vi "RF with WF Sweep plus reference.vi"() -> ()   [LabVIEW 2012]
uses:
  <vilib>/DAQmx/read.llb/DAQmx Read (Counter U32 1Chan 1Samp).vi
  <vilib>/Utility/file.llb/Write To Spreadsheet File (DBL).vi
  <vilib>/DAQmx/miscellaneous.llb/DAQmx Fill In Error Info.vi
  <vilib>/DAQmx/create/channels.llb/DAQmx Create Channel (CI-Count Edges).vi
  <vilib>/DAQmx/create/channels.llb/DAQmx Create Channel (CO-Pulse Generation-Ticks).vi
  <vilib>/DAQmx/configure/timing.llb/DAQmx Timing (Implicit).vi
  <vilib>/DAQmx/configure/timing.llb/DAQmx Timing (Sample Clock).vi
  <resource>/objmgr/daqmx.rc
panel:
  out "Ref":dbl=487.0
  out "Scan":i32=222
  in  "N Scans":i32=100
  out "freq":dbl=349000000.0
  out "RF":dbl=487.0
  out "loop":i32=99
  in  "file path (dialog if empty)":path
  out "Z Position 2":dbl=39.24
  out "Y Position 2":dbl=141.00216667506004
  out "X Position 2":dbl=-28.668339852561274
  in  "CW for tracking":bool
  in  "Y Parameters":T1={"Number of Y Steps"=200, "Max Y (V)"=2.0, "Min Y (V)"=-2.0}
  in  "X":T2={"Number of X Steps"=200, "Max X (V)"=2.0, "Min X (V)"=-2.0}
  in  "Z Position":dbl=39.24
  in  "Y Position":dbl=136.0
  in  "X Position":dbl=-24.0
  in  "Z-track?":bool=TRUE
  out "XY Graph":cluster{dbl[], u32[]}[](graph)
  in  "Freq Max":dbl=350000000.0
  in  "Freq  Step":dbl=1000000.0
  in  "Freq Min":dbl=250000000.0
  in  "power":dbl=-9.0
  in  "stop":bool
  in  "Path to spinapi.dll":path=path "C:/SpinCore/SpinAPI/dll/spinapi64.dll"
  in  "Pulse offset":dbl
  in  "Tau":dbl=5e-07
  in  "RF Pulse":dbl=1e-07
  in  "Rabi Freq":dbl=11750000.0
  in  "MW Delay":dbl=2e-08
  in  "APD signal width":dbl=3e-07
  in  "Signal Delay":dbl=7.6e-07
  in  "AOM Rest time":dbl=1e-06
  in  "AOM Pulse length":dbl=2.5e-06
  in  "N Loop":i32=100000
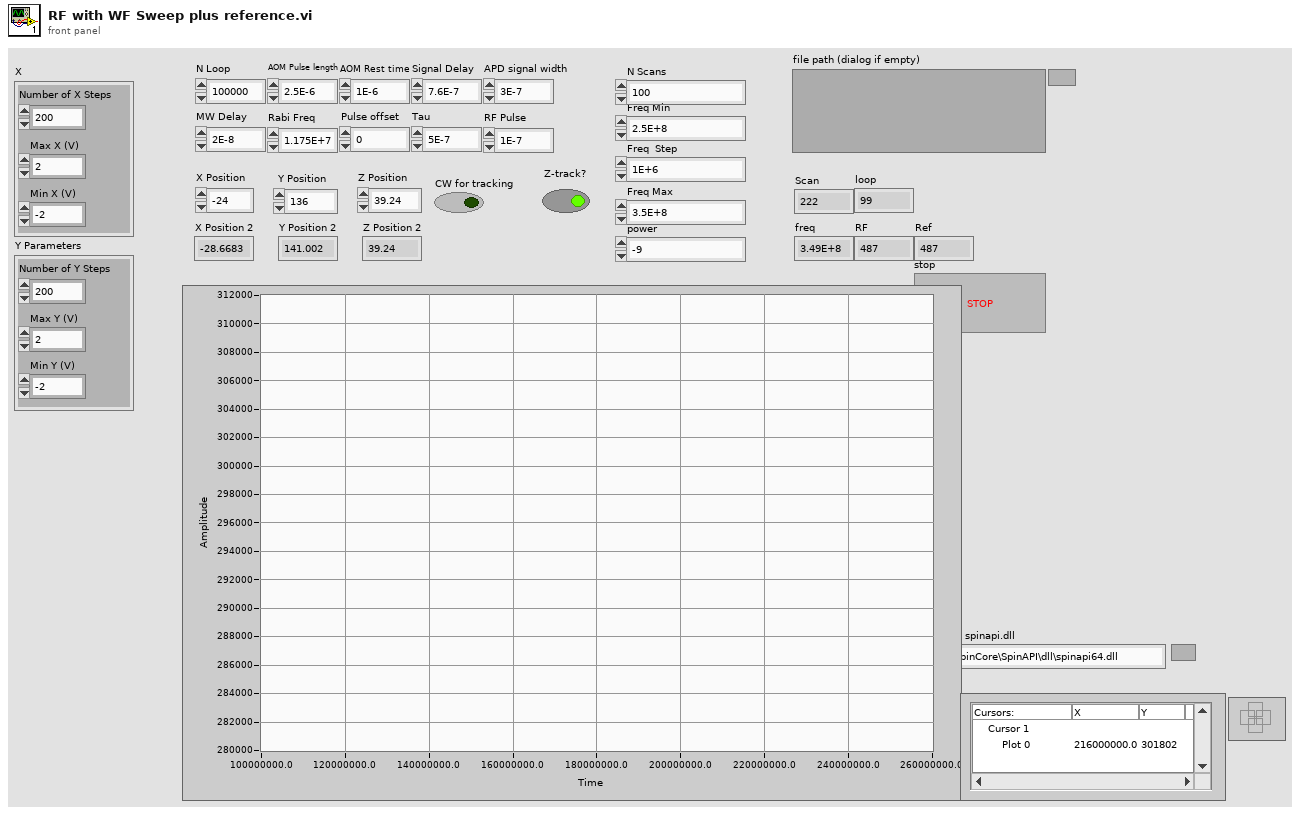
[diagram p1: front panel]
types:
  T1 = cluster{"Number of Y Steps":i32, "Max Y (V)":dbl, "Min Y (V)":dbl}
  T2 = cluster{"Number of X Steps":i32, "Max X (V)":dbl, "Min X (V)":dbl}
  T3 = enum16{"Pulse Program", "Frequency Registers", "TX Phase Registers", "RX Phase Registers"}
  T4 = cluster{"Instruct Data":i32, "Op Code":i32, "Flags":bool[], "Comments":string, "Time (s)":dbl}[]
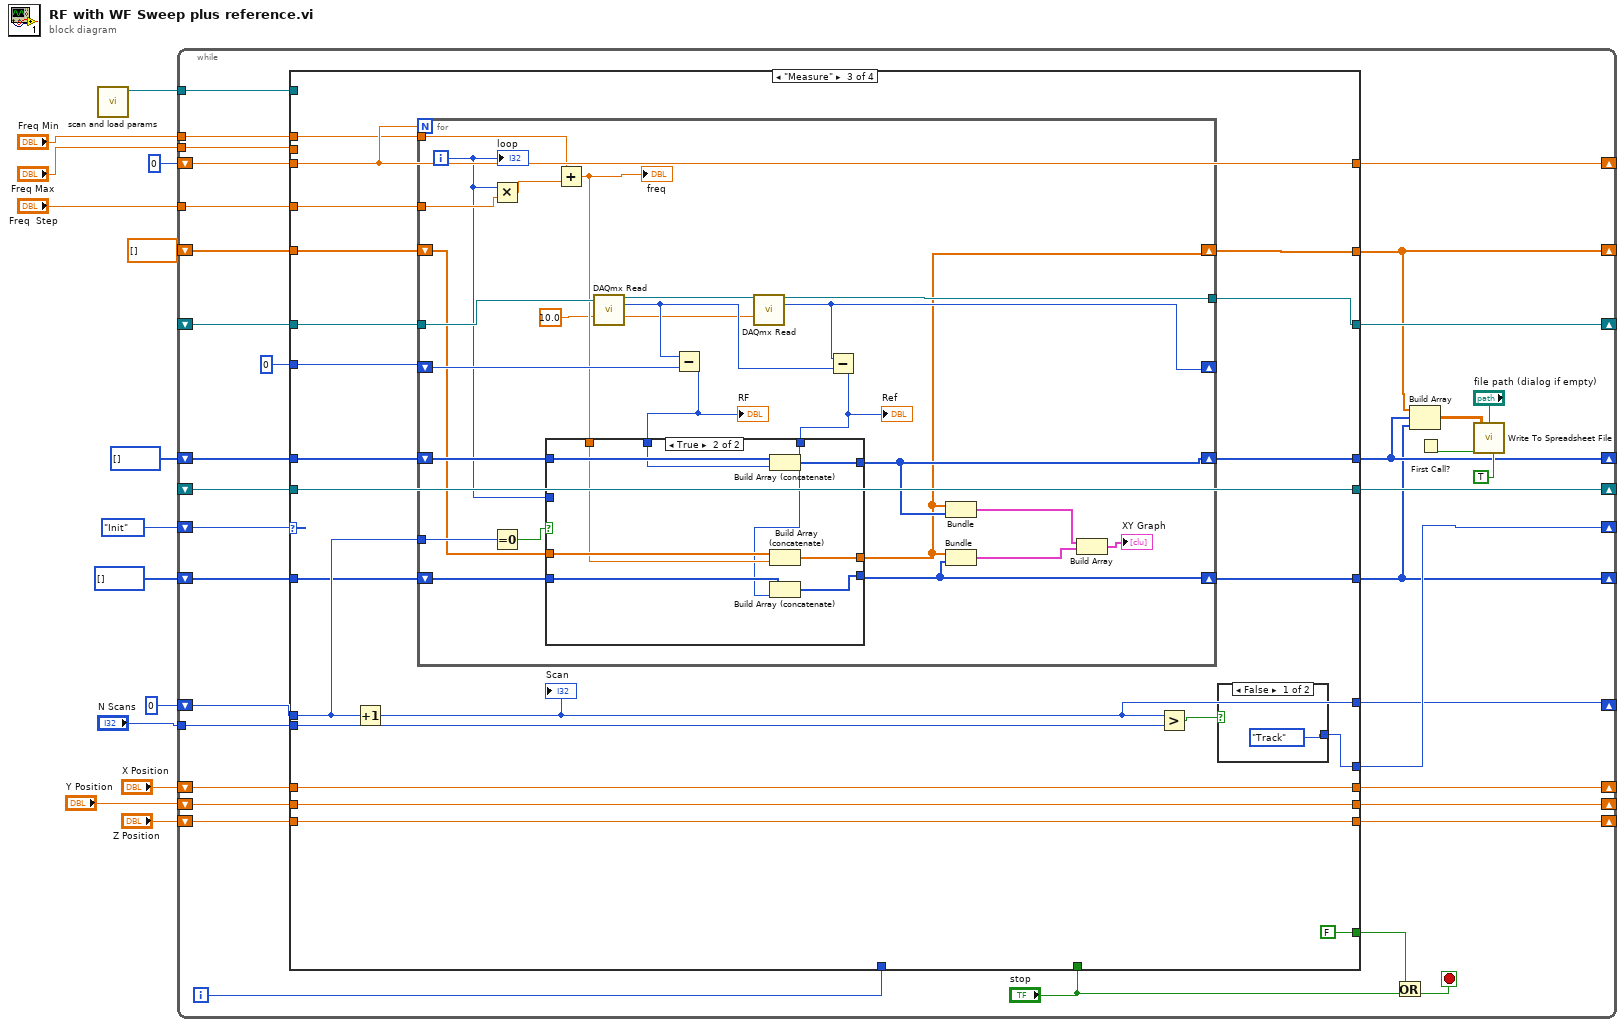
[diagram p0: block diagram]
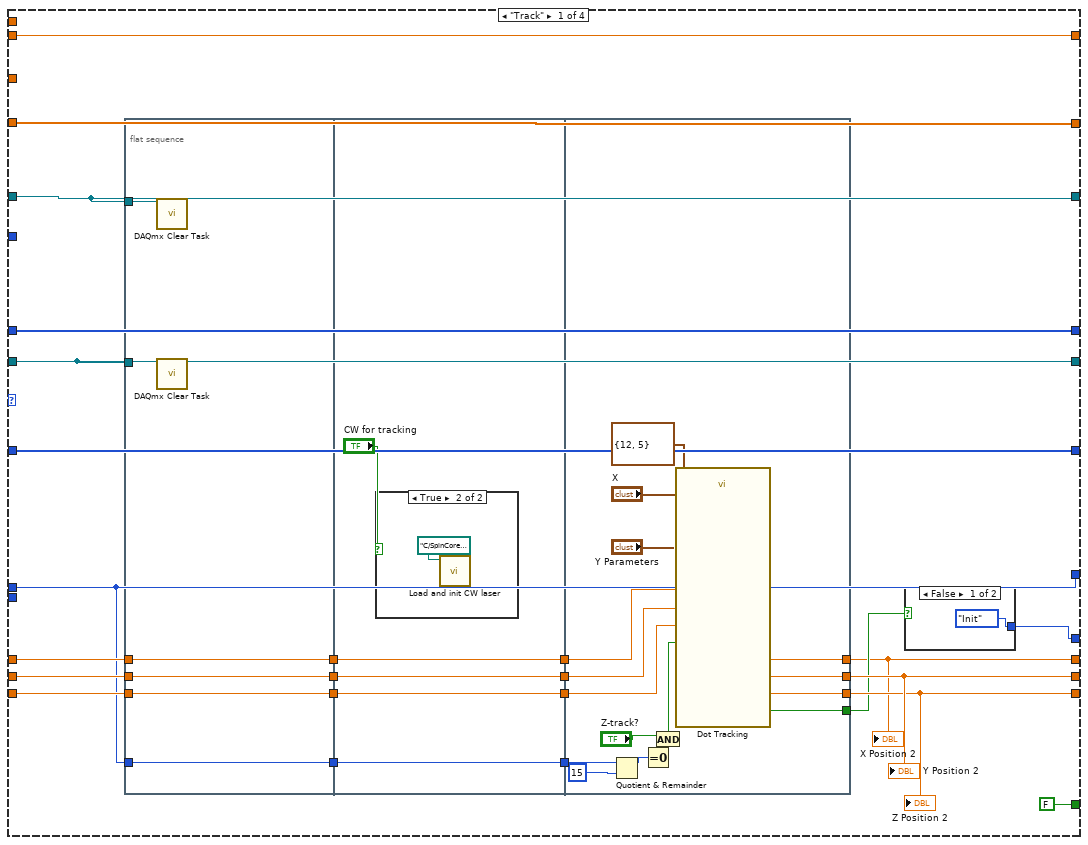
[diagram p2: hidden frame]
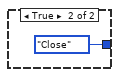
[diagram p3: hidden frame]
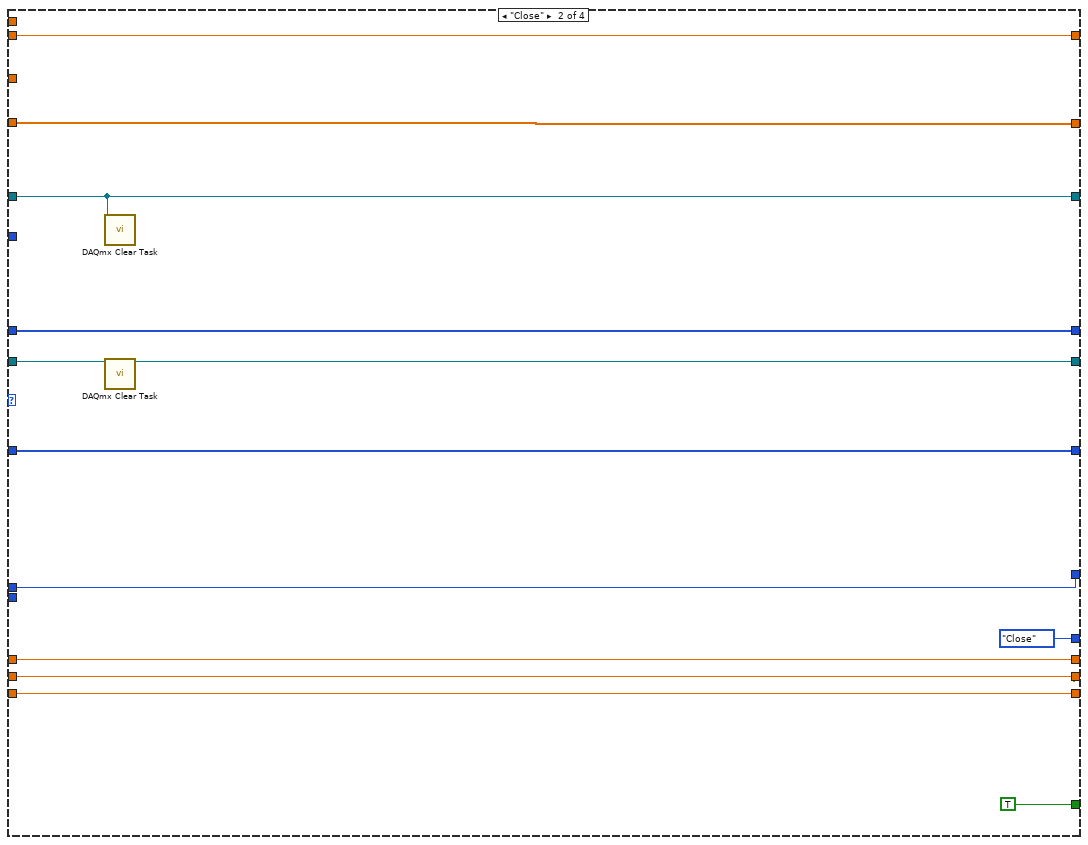
[diagram p5: hidden frame]
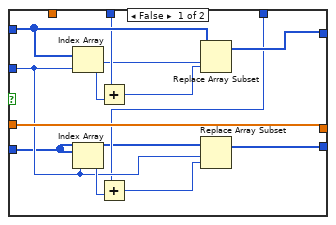
[diagram p6: hidden frame]
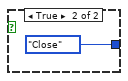
[diagram p7: hidden frame]
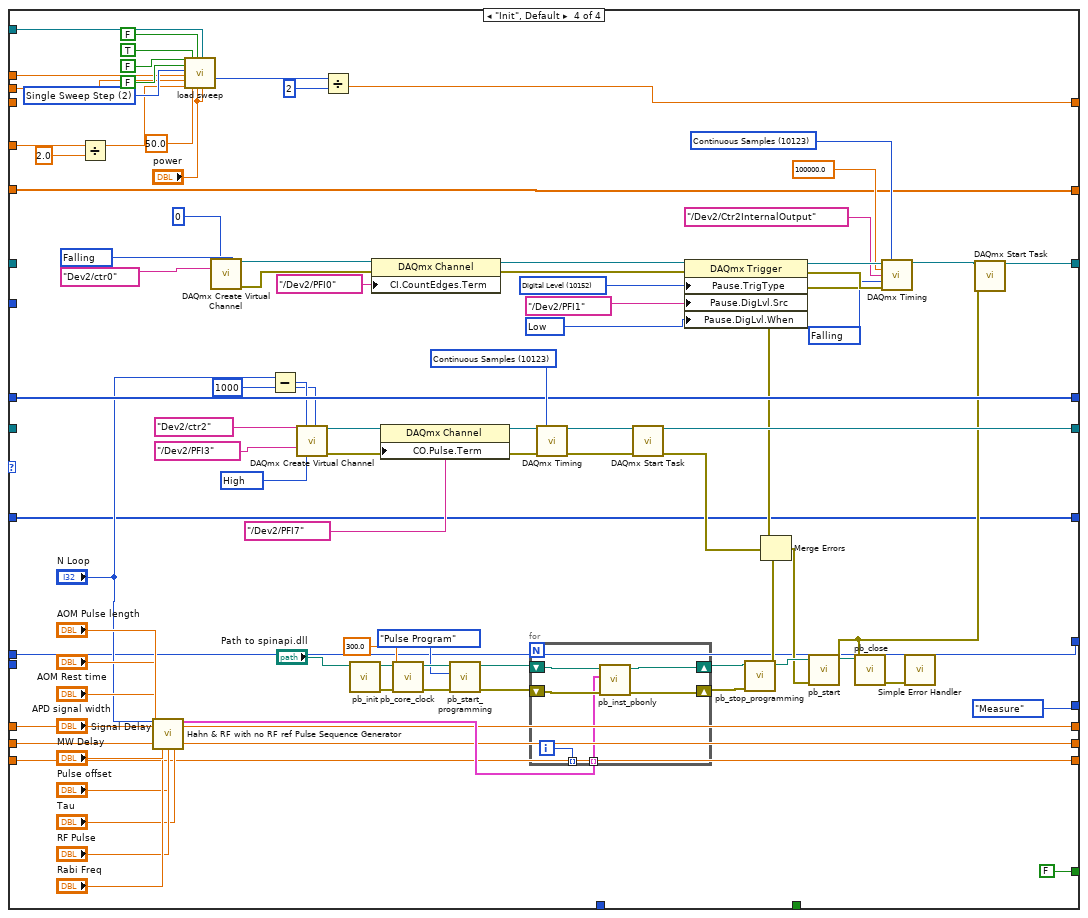
[diagram p8: hidden frame]
diagram:
  n1 = call "scan and load params.vi"() -> ("Serial Port Select"=w8:refnum<visa-resource-name>)  [unwired: 9 out]
  n2 = while {
    shift-right: [w44] -> _
    shift-left: enum16{"Init", "Track", "Measure", "Close", ""}."Init" -> [w50]
    shift-right: [w49] -> _
    shift-left: _ -> [w37]
    shift-right: [w48] -> _
    shift-left: _ -> [w38]
    shift-right: [w19] -> _
    shift-left: u32[] [] -> [w46]
    shift-right: [w32] -> _
    shift-left: dbl[] [] -> [w45]
    shift-right: [w43] -> _
    shift-left: "X Position" -> [w34]
    shift-right: [w42] -> _
    shift-left: "Y Position" -> [w40]
    shift-right: [w41] -> _
    shift-left: "Z Position" -> [w39]
    tunnel: w8 -> [w27]
    tunnel: "Freq  Step" -> [w24]
    tunnel: "Freq Max" -> [w25]
    tunnel: "Freq Min" -> [w26]
    shift-right: [w23] -> _
    shift-left: u16 0 ("Number\nof Points") -> [w22]
    tunnel: "N Scans" -> [w21]
    shift-right: [w18] -> _
    shift-left: 0 -> [w20]
    shift-right: [w15] -> _
    shift-left: u32[] [] -> [w16]
    i -> [w17]
    stop <- w36 stop-if-true
    n3 = case shown="\"Measure\"" w50 {
      tunnel: [w58 w116 w132 w221] -> w49
      tunnel: [w57 w115 w125 w220] -> w48
      tunnel: "stop" -> [_ _ _ _]
      tunnel: w46 -> [w67 w114 w138 w218]
      tunnel: w45 -> [w62 w109 w137 w214]
      tunnel: [w67 w114 w136 w218] -> w19
      tunnel: [w62 w109 w129 w214] -> w32
      tunnel: [w66 enum16{"Init", "Track", "Measure", "Close", ""}."Close" w135 enum16{"Init", "Track", "Measure", "Close", ""}."Measure"] -> w44
      tunnel: [w55 w108 w128 w213] -> w43
      tunnel: [w74 w113 w131 w216] -> w42
      tunnel: [w73 w112 w130 w215] -> w41
      tunnel: w40 -> [w70 w113 w131 w216]
      tunnel: w39 -> [w68 w112 w130 w215]
      tunnel: w38 -> [w57 w115 w133 _]
      tunnel: w37 -> [w58 w116 w132 _]
      tunnel: [FALSE TRUE FALSE FALSE] -> w35
      tunnel: w34 -> [w63 w108 w128 w213]
      tunnel: u32 0 ("data") -> [_ _ w127 _]
      tunnel: w27 -> [_ _ _ w206]
      tunnel: w26 -> [_ _ w124 w198]
      tunnel: w25 -> [_ _ _ w197]
      tunnel: w24 -> [_ _ w123 w196]
      tunnel: [w56 w107 w126 w189] -> w23
      tunnel: w22 -> [w56 w107 w126 _]
      tunnel: w21 -> [_ _ w121 _]
      tunnel: w20 -> [w54 w106 w119 w195]
      tunnel: [w54 w106 w120 w195] -> w18
      tunnel: w17 -> [_ _ _ _]
      tunnel: w16 -> [w51 w105 w118 w192]
      tunnel: [w51 w105 w117 w192] -> w15
      frame "Track" {
        n4 = flat-sequence {
          tunnel: w68 -> [w80]
          tunnel: w70 -> [w81]
          tunnel: w63 -> [w82]
          tunnel: [w82] -> w61
          tunnel: [w81] -> w60
          tunnel: [w80] -> w59
          tunnel: w58 -> [w79]
          tunnel: w57 -> [w78]
          tunnel: w54 -> [w77]
          tunnel: [w77] -> w53
          tunnel: [w87] -> w72
          tunnel: [w86] -> w71
          tunnel: [w85] -> w69
          tunnel: w61 -> [w87]
          tunnel: w60 -> [w86]
          tunnel: w59 -> [w85]
          tunnel: w53 -> [w83]
          tunnel: [w83] -> w52
          tunnel: [w104] -> w55
          tunnel: [w103] -> w74
          tunnel: [w102] -> w73
          tunnel: w72 -> [w101]
          tunnel: w71 -> [w100]
          tunnel: w69 -> [w99]
          tunnel: [w95] -> w65
          tunnel: w52 -> [w89]
          frame #0 {
            n5 = call <vilib>:"DAQmx Clear Task.vi"("task in"=w78) -> ()  [unwired: 14 in, 1 out]
            n6 = call <vilib>:"DAQmx Clear Task.vi"("task in"=w79) -> ()  [unwired: 14 in, 1 out]
          }
          frame #1 {
            n7 = case shown="True" "CW for tracking" {
              frame False {
              }
              frame True {
                n8 = call "Load and init CW laser.vi"("path in"=path "C:/SpinCore/SpinAPI/dll/spinapi64.dll") -> ()  [unwired: 11 in]
              }
            }
          }
          frame #2 {
            n9 = Quotient & Remainder(x=w89, y=15) -> (x-y*floor(x/y)=w93:i32)  [unwired: 1 out]
            n10 = Equal To 0?(x=w93) -> (x = 0?=w92:bool)
            n11 = And(x="Z-track?", y=w92) -> (x .and. y?=w90:bool)
            n12 = call "Dot Tracking.vi"("X"="X", "Y Parameters"="Y Parameters", "RS232 settings"=cluster{"Portnumber":i32, "Baudrate":u16} {"Portnumber"=12, "Baudrate"=5}, "X Pos"=w101, "Y pos"=w100, "Z Pos"=w99, "Z-track?"=w90) -> ("X Position"=w104:dbl, "Y Position"=w103:dbl, "Z Position"=w102:dbl, "Gave up?"=w95:bool)  [unwired: 2 in, 3 out]
          }
        }
        n13 = case shown="False" w65 {
          tunnel: [enum16{"Init", "Track", "Measure", "Close", ""}."Init" enum16{"Init", "Track", "Measure", "Close", ""}."Close"] -> w66
          frame False {
          }
          frame True {
          }
        }
        "X Position 2" <- w55
        "Y Position 2" <- w74
        "Z Position 2" <- w73
      }
      frame "Close" {
        n14 = call <vilib>:"DAQmx Clear Task.vi"("task in"=w115) -> ()  [unwired: 14 in, 1 out]
        n15 = call <vilib>:"DAQmx Clear Task.vi"("task in"=w116) -> ()  [unwired: 14 in, 1 out]
      }
      frame "Measure" {
        n16 = Increment(x=w119) -> (x+1=w120:i32)
        "Scan" <- w120
        n17 = for {
          N: w126 -> [_]
          shift-right: [w145] -> w136
          shift-left: w138 -> [w161]
          shift-right: [w143] -> w129
          shift-left: w137 -> [w153]
          tunnel: w133 -> [w163]
          shift-right: [w149] -> _
          shift-left: w127 -> [w162]
          tunnel: [w150] -> w125
          tunnel: w124 -> [w160]
          tunnel: w123 -> [w159]
          tunnel: w119 -> [w156]
          shift-right: [w142] -> w117
          shift-left: w118 -> [w146]
          i -> [w154]
          w139 = 10.0 ("timeout")
          n18 = Multiply(x=w154, y=w159) -> (x*y=w158:dbl)
          n19 = Equal To 0?(x=w156) -> (x = 0?=w155:bool)
          n20 = Add(x=w160, y=w158) -> (x+y=w152:dbl)
          "freq" <- w152
          n21 = call-poly <vilib>:"DAQmx Read.vi"("task/channels in"=w163, "timeout"=w139) -> ("task out"=w151:refnum<k21>, "data"=w148:u32)  [unwired: 11 in, 1 out]
          n22 = Subtract(x=w148, y=w162) -> (x-y=w157:u32)
          "RF" <- w157
          n23 = call-poly <vilib>:"DAQmx Read.vi"("task/channels in"=w151, "timeout"=w139) -> ("task out"=w150:refnum<k21>, "data"=w149:u32)  [unwired: 11 in, 1 out]
          n24 = Subtract(x=w149, y=w148) -> (x-y=w147:u32)
          "Ref" <- w147
          n25 = case shown="True" w155 {
            tunnel: w161 -> [w175 w184]
            tunnel: [w171 w183] -> w145
            tunnel: w157 -> [w173 w182]
            tunnel: w154 -> [w167 _]
            tunnel: w153 -> [w170 w181]
            tunnel: [w170 w180] -> w143
            tunnel: w152 -> [_ w179]
            tunnel: w147 -> [w166 w177]
            tunnel: w146 -> [w165 w178]
            tunnel: [w164 w176] -> w142
            frame False {
              n26 = Index Array(array=w175, index=w167) -> (element=w174:u32)
              n27 = Index Array(array=w165, index=w167) -> (element=w169:u32)
              n28 = Add(x=w173, y=w174) -> (x+y=w172:u32)
              n29 = Add(x=w166, y=w169) -> (x+y=w168:u32)
              n30 = Replace Array Subset(array=w175, new element=w172, index=w167) -> (w171:u32[])
              n31 = Replace Array Subset(array=w165, new element=w168, index=w167) -> (w164:u32[])
            }
            frame True {
              n32 = Build Array (concatenate)(w184, w182) -> (w183:u32[])
              n33 = Build Array (concatenate)(w181, w179) -> (w180:dbl[])
              n34 = Build Array (concatenate)(w178, w177) -> (w176:u32[])
            }
          }
          n35 = Bundle(w143, w145) -> (w144:cluster{dbl[], u32[]})  [unwired: 1 in]
          n36 = Bundle(w143, w142) -> (w141:cluster{dbl[], u32[]})  [unwired: 1 in]
          n37 = Build Array(w144, w141) -> (→"XY Graph":cluster{dbl[], u32[]}[])
          "loop" <- w154
        }
        n38 = Greater?(x=w120, y=w121) -> (0:w122:bool)
        n39 = case shown="False" w122 {
          tunnel: [enum16{"Init", "Track", "Measure", "Close", ""}."Track" enum16{"Init", "Track", "Measure", "Close", ""}."Close"] -> w135
          frame False {
          }
          frame True {
          }
        }
      }
      frame "Init", Default {
        w193 = 10171 items=["Rising"=10280, "Falling"=10171] ("active edge")
        w194 = 10192 items=["High"=10192, "Low"=10214] ("idle state")
        w201 = 2 items=["No Triggers", "Full Frequency Sweep", "Single Sweep Step", "Stop All", "Digital RF On/Off", "Remove Interrupts", "Reserved 1", "Reserved 2", "Ext AM Modulation", "Ext FM Modulation"] ("Trigger")
        w207 = 1000 ("y")
        w229 = 10123 items=["Finite Samples"=10178, "Continuous Samples"=10123, "Hardware Timed Single Point"=12522] ("sample mode")
        w247 = 10214 items=["High"=10192, "Low"=10214] ("Pause.DigLvl.When")
        w249 = 10152 items=["Analog Level"=10101, "Analog Window"=10103, "Digital Level"=10152, "Digital Pattern"=10398, "None"=10230] ("Pause.TrigType")
        w236 = 10123 items=["Finite Samples"=10178, "Continuous Samples"=10123, "Hardware Timed Single Point"=12522] ("sample mode")
        w225 = 10171 items=["Rising"=10280, "Falling"=10171] ("edge")
        n40 = Divide(x=w196, y=2.0) -> (x/y=w191:dbl)
        n41 = call "Hahn & RF with no RF ref Pulse Sequence Generator.vi"("N Loop"="N Loop", "Rabi Frequency"="Rabi Freq", "RF Pulse"="RF Pulse", "Tau"="Tau", "AOM Pulse length"="AOM Pulse length", "AOM Rest time"="AOM Rest time", "Signal Delay"="Signal Delay", "APD signal width"="APD signal width", "MW Delay"="MW Delay", "Pulse offset"="Pulse offset") -> ("Pulse Sequence"=w250:T4)  [unwired: 5 in]
        n42 = call "load sweep.vi"("Channel"=FALSE, "Sweep\nContinuously"=FALSE ("Sweep\nContinuously"), "Trigger"=w201, "Start Frequency"=w198, "Stop Frequency"=w197, "Step Size MHz"=w191, "RF On"=TRUE, "Step Time (mS)"=50.0, "load?"=FALSE, "Start Amplitude"="power", "Serial Port Select"=w206, "Stop Amplitude"="power") -> ("Number\nof Points"=w188:u16)  [unwired: 7 in]
        n43 = call-poly <vilib>:"DAQmx Create Virtual Channel.vi"("initial count"=u32 0, "edge"=w225, "counter"=tag "Dev2/ctr0") -> ("task out"=w245:refnum<k21>, "error out"=w242:errorcluster)  [unwired: 6 in, 5 out]
        n44 = Subtract(x="N Loop", y=w207) -> (x-y=w209:i32)
        n45 = call-poly <vilib>:"DAQmx Create Virtual Channel.vi"("high ticks"=w209, "low ticks"=w207, "counter"=tag "Dev2/ctr2", "source of ticks"=tag "/Dev2/PFI3" ("source"), "idle state"=w194) -> ("task out"=w233:refnum<k21>, "error out"=w231:errorcluster)  [unwired: 9 in]
        n46 = Divide(x=w188, y=u16 2) -> (x/y=w189:dbl)
        n47 = call "pb_init.vi"("path in"="Path to spinapi.dll") -> ("error out"=w256:errorcluster, "path out"=w254:path)  [unwired: 3 in, 6 out]
        n48 = property class="DAQmx Channel"(reference=w245, error in=w242, "CI.CountEdges.Term"=tag "/Dev2/PFI0") -> (reference out=w246:refnum<k21>, error out=w244:errorcluster)
        n49 = property class="DAQmx Channel"(reference=w233, "CO.Pulse.Term"=tag "/Dev2/PFI7") -> (reference out=w228:refnum<k21>)  [unwired: 1 in, 1 out]
        n50 = call "pb_core_clock.vi"("error in (no error)"=w256, "clock_freq (MHz)"=300.0, "path in"=w254) -> ("error out"=w257:errorcluster, "path out"=w255:path)  [unwired: 7 in]
        n51 = call "pb_start_programming.vi"("error in (no error)"=w257, "Device"=T3."Pulse Program", "path in"=w255) -> ("error out"=w260:errorcluster, "path out"=w259:path)  [unwired: 1 in, 6 out]
        n52 = for {
          shift-right: [w277] -> w261
          shift-left: w259 -> [w279]
          shift-right: [w276] -> w262
          shift-left: w260 -> [w278]
          tunnel: [w275] -> _ mode=indexing
          tunnel: w250 -> [w274] mode=indexing
          i -> [w275]
          n53 = call "pb_inst_pbonly.vi"("error in (no error)"=w278, "PB Instruction"=w274, "path in"=w279) -> ("error out"=w276:errorcluster, "path out"=w277:path)  [unwired: 2 in, 5 out]
        }
        n54 = call-poly <vilib>:"DAQmx Timing.vi"("task/channels in"=w228, "sample mode"=w229, "error in"=w231) -> ("task out"=w232:refnum<k21>, "error out"=w230:errorcluster)  [unwired: 11 in]
        n55 = call <vilib>:"DAQmx Start Task.vi"("task/channels in"=w232, "error in"=w230) -> ("task out"=w221:refnum<k21>, "error out"=w224:errorcluster)  [unwired: 12 in]
        n56 = property class="DAQmx Trigger"(reference=w246, error in=w244, "Pause.TrigType"=w249, "Pause.DigLvl.Src"=tag "/Dev2/PFI1", "Pause.DigLvl.When"=w247) -> (reference out=w241:refnum<k21>, error out=w240:errorcluster)
        n57 = call "pb_stop_programming.vi"("error in (no error)"=w262, "path in"=w261) -> ("error out"=w222:errorcluster, "path out"=w252:path)  [unwired: 1 in, 7 out]
        n58 = call-poly <vilib>:"DAQmx Timing.vi"("task/channels in"=w241, "sample mode"=w236, "rate"=100000.0, "source"=tag "/Dev2/Ctr2InternalOutput", "active edge"=w193, "error in"=w240) -> ("task out"=w238:refnum<k21>, "error out"=w211:errorcluster)  [unwired: 8 in]
        n59 = Merge Errors(w211, w224, w222) -> (w223:errorcluster)
        n60 = call "pb_start.vi"("error in (no error)"=w223, "path in"=w252) -> ("error out"=w210:errorcluster, "path out"=w251:path)  [unwired: 1 in, 7 out]
        n61 = call "pb_close.vi"("error in (no error)"=w210, "path in"=w251) -> ("error out"=w264:errorcluster)  [unwired: 9 out]
        n62 = call <vilib>:"Simple Error Handler.vi"("error in (no error)"=w264) -> ()  [unwired: 1 in, 8 out]
        n63 = call <vilib>:"DAQmx Start Task.vi"("task/channels in"=w238, "error in"=w210) -> ("task out"=w220:refnum<k21>)  [unwired: 13 out]
      }
    }
    n64 = Or(x=w35, y="stop") -> (x .or. y?=w36:bool)
    n65 = Build Array(w32, w19, w15) -> (w31:dbl[][])
    n66 = First Call?() -> (First Call?: T/F=w28:bool)
    n67 = call-poly <vilib>:"Write To Spreadsheet File.vi"("transpose? (no:F)"=TRUE, "append to file? (new file:F)"=w28, "2D data"=w31, "file path (dialog if empty)"="file path (dialog if empty)") -> ()  [unwired: 4 in, 1 out]
  }
